vi "create_image_names_file.vi"(7 "force format?":T1=enum."uint8", 8 "error in (no error)":errorcluster, 9 "file path in (can be empty)":path, 11 "ImageCollection in":refnum<class "ImageCollection.lvclass">) -> (0 "error out":errorcluster, 1 "file path out":path, 3 "ImageCollection out":refnum<class "ImageCollection.lvclass">)   [LabVIEW 2010, in "ImageCollection.lvclass"]
uses:
  ImageCollection.lvclass
  Image/Image/target_format_enum.ctl
  Image/Image/Image.lvclass
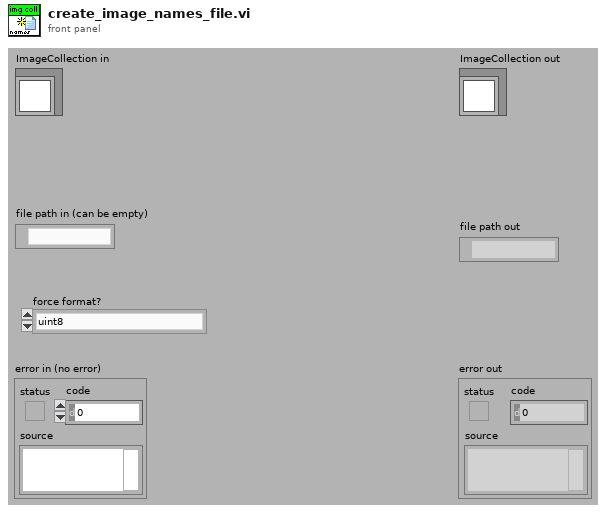
[diagram p1: front panel]
types:
  T1 = typedef "target_format_enum.ctl" = enum16{"don't force", "uint8", "uint16", "int16", "uint32", "int32", "single float"}
  T2 = enum16{"open", "replace", "create", "open or create", "replace or create", "replace or create with confirmation"}
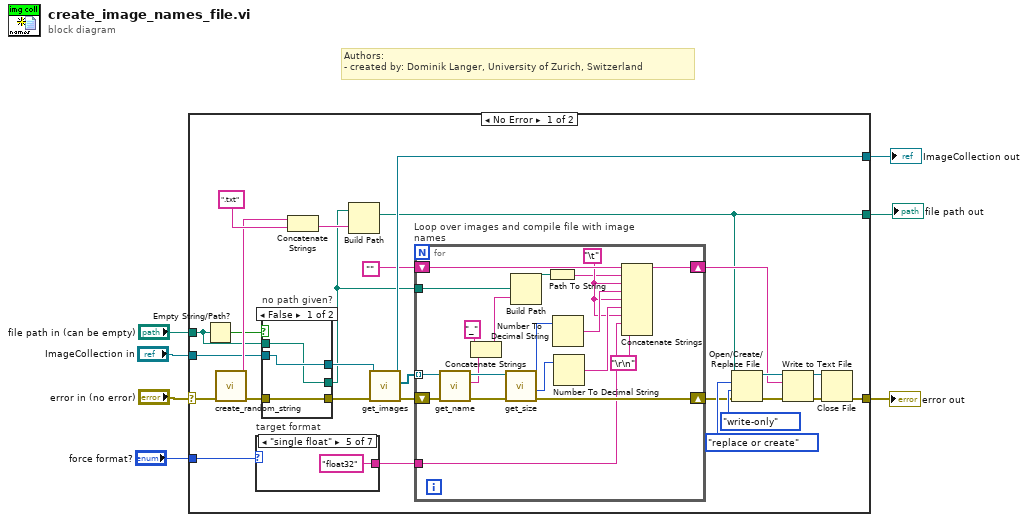
[diagram p0: block diagram]
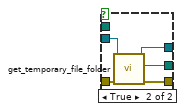
[diagram p2: hidden frame]
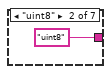
[diagram p4: hidden frame]
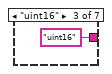
[diagram p5: hidden frame]
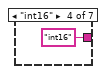
[diagram p6: hidden frame]
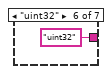
[diagram p7: hidden frame]
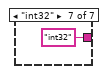
[diagram p8: hidden frame]
diagram:
  # "Authors: \n- created by: Dominik Langer, University of Zurich, Switzerland"
  n1 = case shown="No Error" "error in (no error)" {
    selector: "error in (no error)" -> [w27 w70]
    tunnel: [w26 w70] -> w6
    tunnel: [w23 w69] -> w4
    tunnel: "ImageCollection in" -> [w24 w69]
    tunnel: [w14 _] -> w3
    tunnel: "force format?" -> [w11 _]
    tunnel: "file path in (can be empty)" -> [w8 _]
    frame No Error {
      n2 = Empty String/Path?(string/path=w8) -> (empty?=w9:bool)
      n3 = call "create_random_string.vi"("error in (no error)"=w27) -> ("error out"=w28:errorcluster, "random string"=w25:string)  [unwired: 1 in, 8 out]
      n4 = case "target format" shown="\"single float\"" w11 {
        tunnel: [_ "uint8" ("string") "uint16" ("string") "int16" ("string") "float32" ("string") "uint32" ("string") "int32" ("string")] -> w10
        frame "don't force", Default {
        }
        frame "uint8" {
        }
        frame "uint16" {
        }
        frame "int16" {
        }
        frame "single float" {
        }
        frame "uint32" {
        }
        frame "int32" {
        }
      }
      n5 = case "no path given?" shown="False" w9 {
        tunnel: [w36 w42] -> w31
        tunnel: w28 -> [w37 w41]
        tunnel: w24 -> [w36 w40]
        tunnel: [w37 w39] -> w16
        tunnel: [w35 w38] -> w12
        tunnel: w8 -> [w35 _]
        frame False {
        }
        frame True {
          n6 = call-dynamic "get_temporary_file_folder.vi"("error in (no error)"=w41, "ImageCollection.lvclass in"=w40) -> ("error out"=w39:errorcluster, "temporary file folder"=w38:path, "ImageCollection.lvclass out"=w42:refnum<class "ImageCollection.lvclass">)  [unwired: 7 out]
        }
      }
      n7 = Concatenate Strings(w25, ".txt" ("string")) -> (w22:string)
      n8 = Build Path(base path=w12, name or relative path=w22) -> (appended path=w14:path)
      n9 = call-dynamic "get_images.vi"("error in (no error)"=w16, "ImageCollection.lvclass in"=w31) -> ("error out"=w34:errorcluster, "images"=w33:refnum<class "Image.lvclass">[], "ImageCollection.lvclass out"=w23:refnum<class "ImageCollection.lvclass">)  [unwired: 7 out]
      n10 = for "Loop over images and compile file with image names" {
        shift-right: [w54] -> w19
        shift-left: w34 -> [w66]
        tunnel: w33 -> [w65] mode=indexing
        shift-right: [w68] -> w15
        shift-left: "" -> [w67]
        tunnel: w12 -> [w64]
        tunnel: w10 -> [w53]
        w56 = "\t"
        n11 = call-dynamic "get_name.vi"("error in (no error)"=w66, "Image in"=w65) -> ("error out"=w62:errorcluster, "name"=w50:string, "Image out"=w61:refnum<class "Image.lvclass">)  [unwired: 7 out]
        n12 = Concatenate Strings("_" ("string"), w50) -> (w49:string)
        n13 = call-dynamic "get_size.vi"("error in (no error)"=w62, "Image in"=w61) -> ("error out"=w54:errorcluster, "y resolution"=w59:i32, "x resolution"=w60:i32)  [unwired: 7 out]
        n14 = Build Path(base path=w64, name or relative path=w49) -> (appended path=w63:path)
        n15 = Path To String(path=w63) -> (string=w51:string)
        n16 = Number To Decimal String(number=w60) -> (decimal integer string=w58:string)  [unwired: 1 out]
        n17 = Number To Decimal String(number=w59) -> (decimal integer string=w57:string)  [unwired: 1 out]
        n18 = Concatenate Strings(w67, w51, w56, w58, w56, w57, w56, w53, "\r\n") -> (w68:string)
      }
      n19 = Open/Create/Replace File(file path (use dialog)=w14, error in=w19, operation (0:open)=T2."replace or create", access (0:read/write)=enum16{"read/write", "read-only", "write-only"}."write-only") -> (refnum out=w17:refnum<file>, error out=w18:errorcluster)  [unwired: 3 out]
      n20 = Write to Text File(file (use dialog)=w17, text=w15, error in=w18) -> (refnum out=w20:refnum<file>, error out=w21:errorcluster)  [unwired: 2 out]
      n21 = Close File(refnum=w20, error in=w21) -> (error out=w26:errorcluster)  [unwired: 1 out]
    }
    frame Error {
    }
  }
  "error out" <- w6
  "ImageCollection out" <- w4
  "file path out" <- w3
